vi "Read Value by Name.vi"(8 "error in (no error)":errorcluster, 10 "Data Name":string, 11 "Current Value Table":T1) -> (0 "error out":errorcluster, 1 "Value Found?":bool, 2 "Current Value":variant, 3 "Current Value Table":T1)   [LabVIEW 2015, in "CurrentValueTable.lvlib" / "CurrentValueTable.lvclass"]
uses:
  CurrentValueTable.lvclass
  CurrentValueTable Reference.ctl
  CurrentValueTable.lvclass/CurrentValueTable.ctl
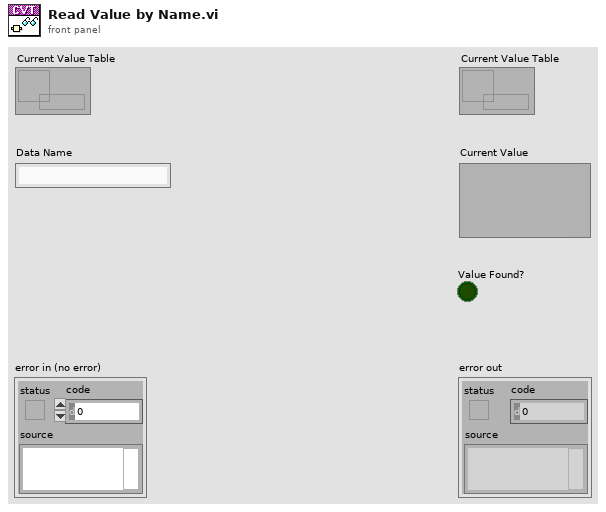
[diagram p1: front panel]
types:
  T1 = typedef "CurrentValueTable.lvlib/CurrentValueTable.lvclass/CurrentValueTable Reference.ctl" = refnum<data-value>
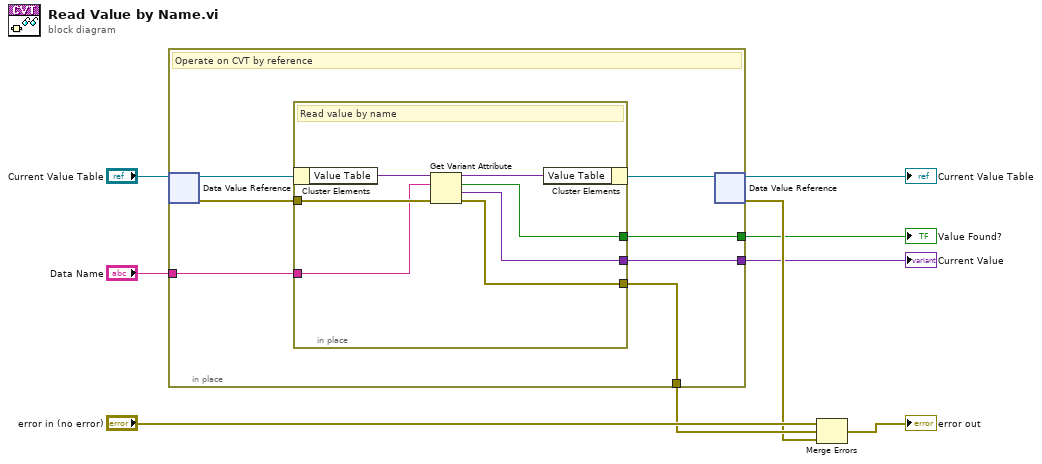
[diagram p0: block diagram]
diagram:
  n1 = in-place {
    in-place-border: [w13] -> w5
    in-place-border: "Data Name" -> [w12]
    in-place-border: [w16] -> w2
    in-place-border: [w10] -> w1
    # "Operate on CVT by reference"
    n2 = in-place-dvr #1("Current Value Table") -> (w15:refnum<class "CurrentValueTable.lvclass">, w11:errorcluster)
    n3 = in-place {
      in-place-border: w11 -> [w23]
      in-place-border: [w22] -> w13
      in-place-border: w12 -> [w21]
      in-place-border: [w18] -> w16
      in-place-border: [w17] -> w10
      # "Read value by name"
      n4 = in-place-cluster #2(w15) -> ("Value Table"=w20:variant)
      n5 = Get Variant Attribute(Variant=w20, name=w21, error in=w23) -> (duplicate Variant=w19:variant, found=w17:bool, value=w18:variant, error out=w22:errorcluster)  [unwired: 1 in]
      n6 = in-place-cluster #2("Value Table"=w19) -> (w14:refnum<class "CurrentValueTable.lvclass">)
    }
    n7 = in-place-dvr #1(w14) -> (→"Current Value Table":T1, w4:errorcluster)
  }
  "Current Value" <- w2
  "Value Found?" <- w1
  n8 = Merge Errors("error in (no error)", w5, w4) -> (→"error out":errorcluster)
